vi "galilDR_Parser.vi"() -> ()   [LabVIEW 2015]
panel:
  in  "Boolean":bool=TRUE
  out "*(type *) &x":u16=28640
  out "size(s)":i32=116
  out "byte array":u8[](array[numeric])=[76, 204, 106, 148, 248, 76, 0, 80, 76, 64, 66, 206, 8, 0, 69, 0, 0, 102, 0, 214, 64, 0, 128, 17, 115, 212, 192, 168, 2, 30, 192, 168, 2, 110, 234, 103, 247, 135, 0, 82, 83, 135, 135, 1, 74, 0, 224, 111, 255, 0, 0, 0, 0, 0, 0, 0, 0, 0, 0, 0, 0, 0, 0, 0, 0, 0, 0, 0, 255, 1, 0, 0, 0, 64, 0, 0, 0, 0, 31, 0, 0, 64, 110, 1, 0, 0, 0, 0, 0, 0, 0, 0, 0, 0, 0, 0, 0, 0, 0, 0, 0, 0, 0, 0, 0, 0, 0, 0, 0, 0, 7, 0, 0, 0, 0, 0] format="%.0x"
  in  "Raw Data":string="LÌj”øL\u0000PL@BÎ\b\u0000E\u0000\u0000f\u0000Ö@\u0000€\u0011sÔÀ¨\u0002\u001eÀ¨\u0002nêg÷‡\u0000RS‡‡\u0001J\u0000àoÿ\u0000\u0000\u0000\u0000\u0000\u0000\u0000\u0000\u0000\u0000\u0000\u0000\u0000\u0000\u0000\u0000\u0000\u0000\u0000ÿ\u0001\u0000\u0000\u0000@\u0000\u0000\u0000\u0000\u001f\u0000\u0000@n\u0001\u0000\u0000\u0000\u0000\u0000\u0000\u0000\u0000\u0000\u0000\u0000\u0000\u0000\u0000\u0000\u0000\u0000\u0000\u0000\u0000\u0000\u0000\u0000\u0000\u0000\u0000\u0007\u0000\u0000\u0000\u0000\u0000"
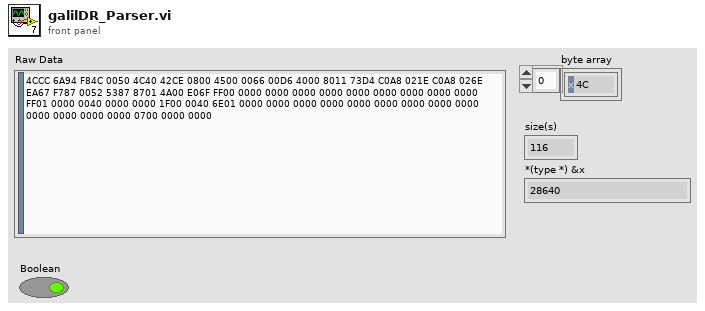
[diagram p1: front panel]
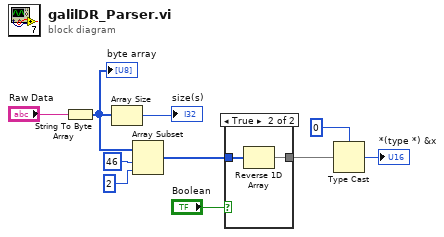
[diagram p0: block diagram]
diagram:
  n1 = String To Byte Array(string="Raw Data") -> (unsigned byte array=w8:u8[])
  "byte array" <- w8
  n2 = Array Size(array=w8) -> (size(s)=→"size(s)":i32)
  n3 = Array Subset(array=w8, index=46, length=2) -> (w3:u8[])
  n4 = case shown="True" "Boolean" {
    tunnel: w3 -> [w11 w12]
    tunnel: [w11 w13] -> w2
    frame False {
    }
    frame True {
      n5 = Reverse 1D Array(array=w12) -> (reversed array=w13:u8[])
    }
  }
  n6 = Type Cast(type=u16 0, x=w2) -> (*(type *) &x=→"*(type *) &x":u16)
